vi "Event Nested Status.vi"(11 "Queue Actor in":refnum<class "Queue Actor.lvclass">) -> (0 "Event Nested Count":i32, 1 "Event Nested Aliases":string[](array[string]), 2 "Any Exist?":bool)   [LabVIEW 2021, in "jettl.lvlib" / "Queue Actor.lvclass"]
uses:
  Queue Actor.lvclass
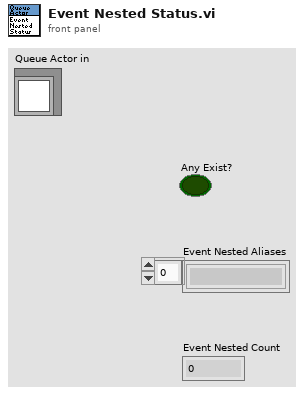
[diagram p1: front panel]
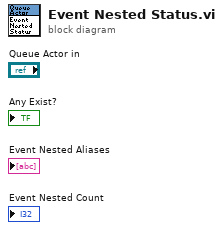
[diagram p0: block diagram]
diagram:
